vi "Basic Generate LV Icon Text Layer.vi"(8 "error in (no error)":errorcluster) -> (0 "error out":errorcluster, 2 "Picture":picture, 3 "Icon.lvlclass out":refnum<class "Icon.lvclass">)   [LabVIEW 2020, in "LabVIEW Icon API.lvlib"]
doc: "Basic example that shows how to set the Text Layer"
uses:
  LabVIEW Icon API.lvlib
  lv_icon/Classes/Icon/Icon.lvclass
  API_Rectangle Dimension.ctl
  API_Text.ctl
  <vilib>/picture/picture.llb/imagedata.ctl
  <vilib>/Utility/miscctls.llb/LVPoint32TypeDef.ctl
  API_User Layer Data.ctl
panel:
  in  "Layer name":string="Circle"
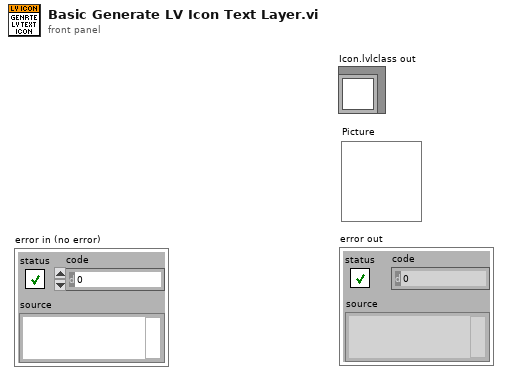
[diagram p1: front panel]
types:
  T1 = cluster{"left":i16, "top":i16, "right":i16, "bottom":i16}
  T2 = typedef "LabVIEW Icon API.lvlib/API_User Layer Data.ctl" = cluster{"Layer name":string, "Origin":T3, "Icon image data":T4}
  T3 = typedef "LVPoint32TypeDef.ctl" = cluster{"Horizontal":i32, "Vertical":i32}
  T4 = typedef "imagedata.ctl" = cluster{"image type":i32, "image depth":i32, "image":u8[], "mask":u8[], "colors":u32[], "Rectangle":cluster{"left":i16, "top":i16, "right":i16, "bottom":i16}}
  T5 = typedef "LabVIEW Icon API.lvlib/API_Text.ctl" = cluster{"Line 1 text":string, "Line 2 text":string, "Line 3 text":string, "Line 4 text":string}
  T6 = typedef "LabVIEW Icon API.lvlib/API_Rectangle Dimension.ctl" = cluster{"Width":i16, "Height":i16}
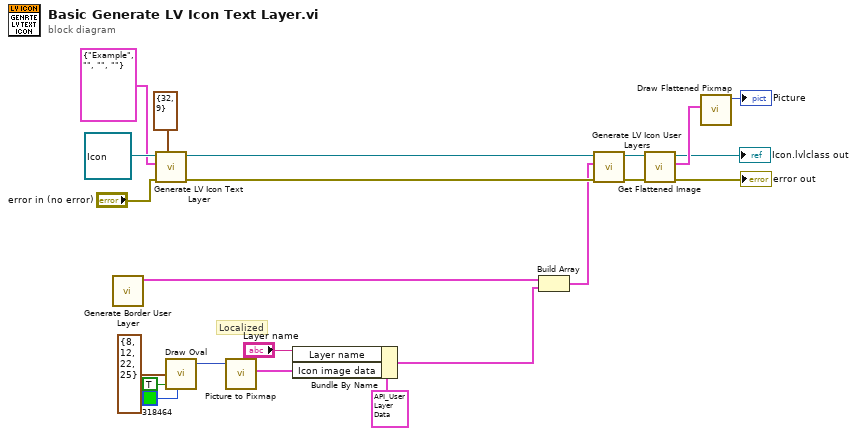
[diagram p0: block diagram]
diagram:
  # "Localized"
  n1 = call "Generate Border User Layer.vi"() -> ("User Layer data"=w5:T2)  [unwired: 11 in]
  n2 = call "Generate LV Icon Text Layer.vi"("Rectangle dimension (32,32)"=T6 {"Width"=32, "Height"=9}, "error in (no error)"="error in (no error)", "Text"=T5 {"Line 1 text"="Example", "Line 2 text"="", "Line 3 text"="", "Line 4 text"=""}, "Icon in"=refnum<class "Icon.lvclass"> refnum ("Icon.lvclass in")) -> ("error out"=w18:errorcluster, "Icon out"=w17:refnum<class "Icon.lvclass">)  [unwired: 6 in]
  n3 = call <vilib>:"Draw Oval.vi"("rect"=T1 {"left"=8, "top"=12, "right"=22, "bottom"=25}, "fill?(F)"=TRUE, "color(black)"=u32 318464) -> ("new picture"=w10:picture)  [unwired: 6 in]
  n4 = call <vilib>:"Picture to Pixmap.vi"("picture"=w10) -> ("image data"=w8:T4)  [unwired: 9 in, 1 out]
  n5 = Bundle By Name(cluster=T2 {"Layer name"="", "Origin"={"Horizontal"=0, "Vertical"=0}, "Icon image data"={"image type"=0, "image depth"=0, "image"=[], "mask"=[], "colors"=[], "Rectangle"={"left"=0, "top"=0, "right"=0, "bottom"=0}}} ("User layer"), "Layer name"="Layer name", "Icon image data"=w8) -> (w4:T2)
  n6 = Build Array(w5, w4) -> (w3:T2[])
  n7 = call "Generate LV Icon User Layers.vi"("error in (no error)"=w18, "User layers"=w3, "Icon in"=w17) -> ("error out"=w15:errorcluster, "Icon out"=w6:refnum<class "Icon.lvclass">)  [unwired: 7 in]
  n8 = call "Get Flattened Image.vi"("error in (no error)"=w15, "lv_icon.lvlib:Icon.lvclass in"=w6) -> ("error out"=→"error out":errorcluster, "Color Image"=w19:T4, "lv_icon.lvlib:Icon.lvclass out"=→"Icon.lvlclass out":refnum<class "Icon.lvclass">)  [unwired: 6 in, 1 out]
  n9 = call <vilib>:"Draw Flattened Pixmap.vi"("image data"=w19) -> ("new picture"=→"Picture":picture)  [unwired: 8 in]
